vi "test- popup new messages.vi"(8 "error in (no error)":errorcluster, 11 "TestCase in":refnum<class "testcase-csm loop support.lvclass">) -> (0 "error out":errorcluster, 3 "TestCase out":refnum<class "testcase-csm loop support.lvclass">)   [LabVIEW 2017, in "testcase-csm loop support.lvclass"]
uses:
  testcase-csm loop support.lvclass
  <vilib>/addons/_JKI Toolkits/VI Tester/TestCase.llb/TestCase.lvclass
  src/user.lib/_NEVSTOP/Communicable State Machine(CSM)/addons/Loop-Support/CSM Loop Support.lvlib
  src/user.lib/_NEVSTOP/Communicable State Machine(CSM)/Communicable State Machine.lvlib
  C:/Program Files (x86)/National Instruments/LabVIEW 2017/vi.lib/addons/_JKI Toolkits/VI Tester/TestCase.llb/TestCase.lvclass
panel:
  out "expected result":string="dosth2\ndosth3\naction: check -><loop>\ndosth1\naction: end -><end>\nPostSendMsg >>  1122 -& caller >>>> api >> arg"
  out "Remaining States":string
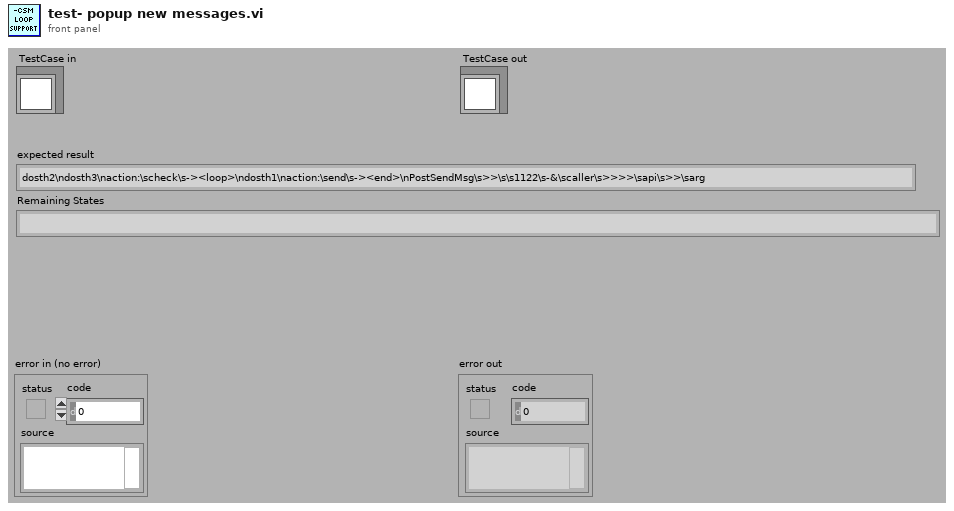
[diagram p1: front panel]
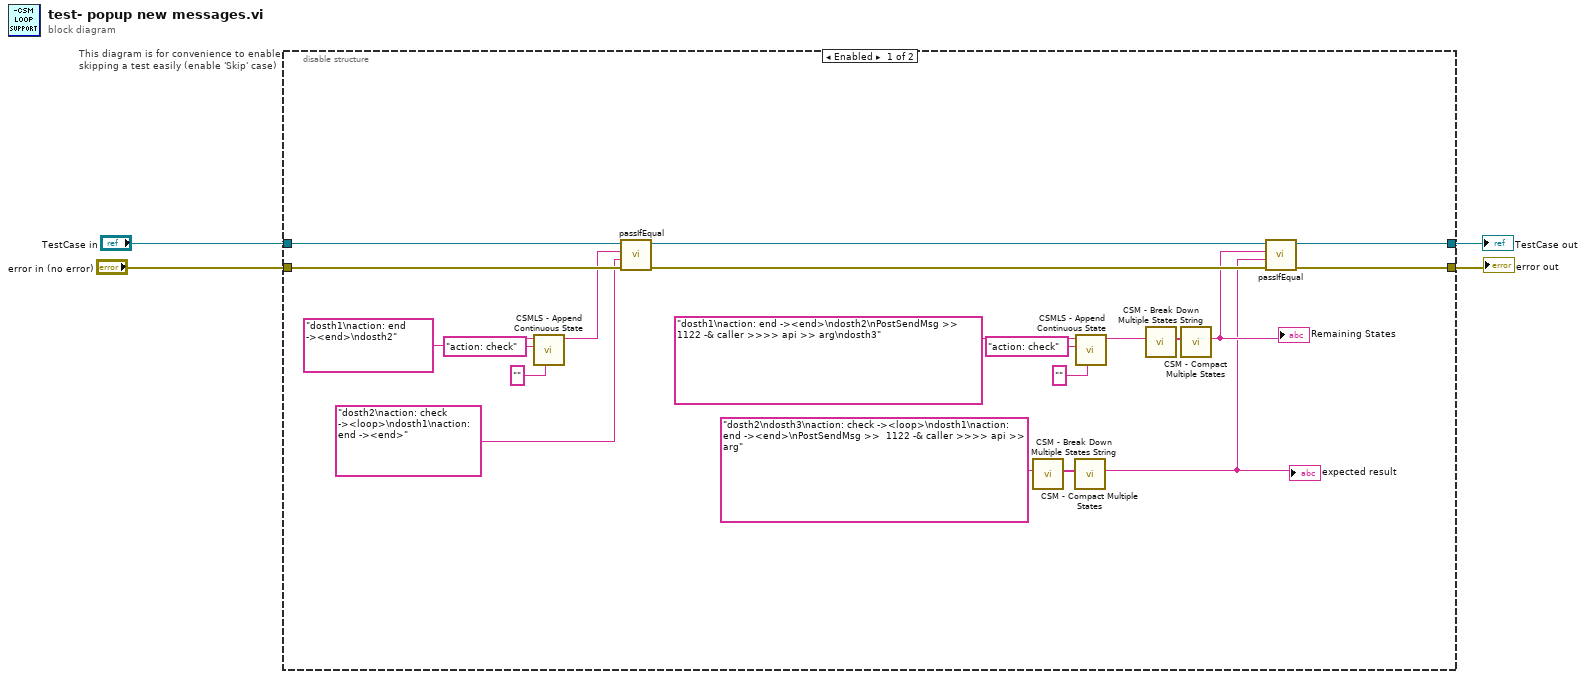
[diagram p0: block diagram]
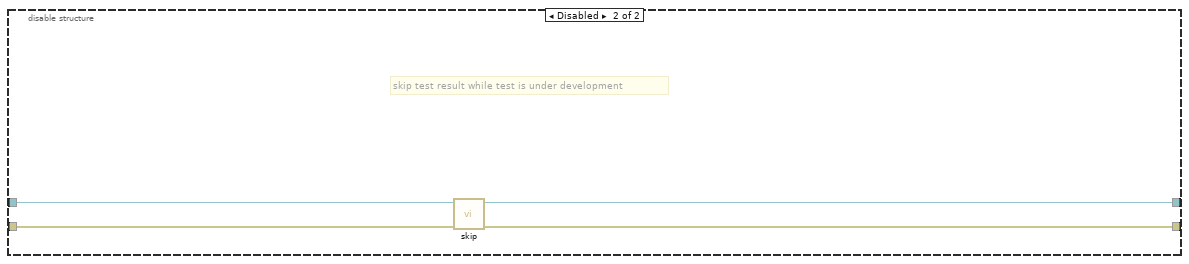
[diagram p2: hidden frame]
diagram:
  n1 = disable-structure "This diagram is for convenience to enable skipping a test easily (enable 'Skip' case)" shown="Enabled" {
    disable-tunnel: "TestCase in" -> [w24 w28]
    disable-tunnel: [w11 w26] -> w1
    disable-tunnel: [w12 w27] -> w3
    disable-tunnel: "error in (no error)" -> [w23 w25]
    frame Enabled {
      n2 = call "CSMLS - Append Continuous State.vi"("Loop State(s) And Arguments"="" ("Loop State(s) and Arguments"), "Continous State"="action: check", "States Queue"="dosth1\naction: end -><end>\ndosth2" ("expected result")) -> ("Remaining States"=w21:string)  [unwired: 8 in]
      n3 = call-dynamic "passIfEqual.vi"("error in (no error)"=w23, "y"="dosth2\naction: check -><loop>\ndosth1\naction: end -><end>" ("expected result"), "x"=w21, "TestCase in"=w24) -> ("error out"=w9:errorcluster, "TestCase out"=w10:refnum<class "testcase-csm loop support.lvclass">)  [unwired: 6 in]
      n4 = call "CSM - Break Down Multiple States String.vi"("States"="dosth2\ndosth3\naction: check -><loop>\ndosth1\naction: end -><end>\nPostSendMsg >>  1122 -& caller >>>> api >> arg" ("expected result")) -> ("Multiple States"=w7:string[])  [unwired: 10 in]
      n5 = call "CSM - Compact Multiple States.vi"("Multiple States"=w7) -> ("States"=w5:string)  [unwired: 9 in]
      "expected result" <- w5
      n6 = call "CSMLS - Append Continuous State.vi"("Loop State(s) And Arguments"="" ("Loop State(s) and Arguments"), "Continous State"="action: check", "States Queue"="dosth1\naction: end -><end>\ndosth2\nPostSendMsg >>  1122 -& caller >>>> api >> arg\ndosth3" ("expected result")) -> ("Remaining States"=w14:string)  [unwired: 8 in]
      n7 = call "CSM - Break Down Multiple States String.vi"("States"=w14) -> ("Multiple States"=w8:string[])  [unwired: 10 in]
      n8 = call "CSM - Compact Multiple States.vi"("Multiple States"=w8) -> ("States"=w6:string)  [unwired: 9 in]
      "Remaining States" <- w6
      n9 = call-dynamic "passIfEqual.vi"("error in (no error)"=w9, "y"=w5, "x"=w6, "TestCase in"=w10) -> ("error out"=w12:errorcluster, "TestCase out"=w11:refnum<class "testcase-csm loop support.lvclass">)  [unwired: 6 in]
    }
    frame Disabled {
      # "skip test result while test is under development"
      n10 = call <vilib>:"skip.vi"("error in (no error)"=w25, "TestCase in"=w28) -> ("error out"=w27:errorcluster, "TestCase out"=w26:refnum<class "testcase-csm loop support.lvclass">)  [unwired: 8 in]
    }
  }
  "error out" <- w3
  "TestCase out" <- w1
